vi "Calculate Ball Trajectory.vi"() -> ()   [LabVIEW 2013]
panel:
  in  "Ball Data":T1
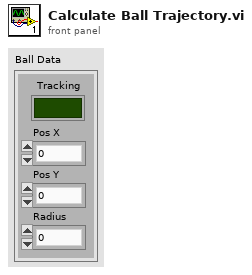
[diagram p1: front panel]
types:
  T1 = cluster{"Tracking":bool, "Pos X":dbl, "Pos Y":dbl, "Radius":dbl}
  T2 = cluster{bool, "Numeric":dbl, "Numeric":dbl, "Numeric":dbl}
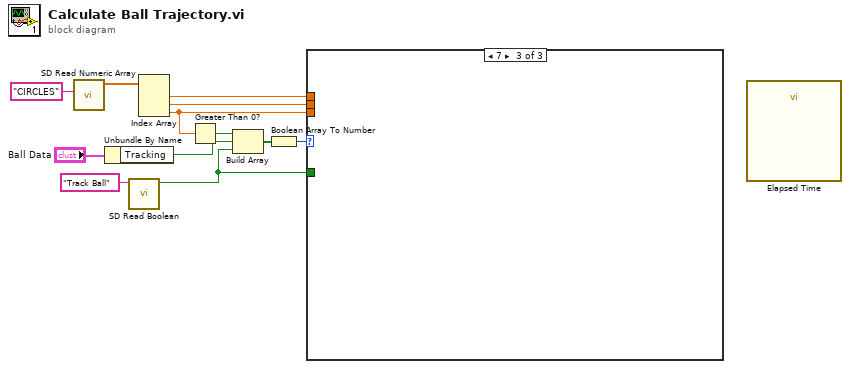
[diagram p0: block diagram]
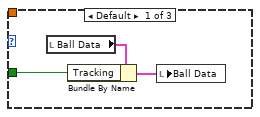
[diagram p2: hidden frame]
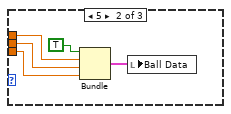
[diagram p3: hidden frame]
diagram:
  n1 = call <vilib>:"SD Read Numeric Array.vi"("Table Prefix"="CIRCLES") -> ("Numeric Array"=w10:dbl[])  [unwired: 8 in, 2 out]
  n2 = Unbundle By Name("Ball Data") -> ("Tracking"=w8:bool)
  n3 = call <vilib>:"SD Read Boolean.vi"("Name"="Track Ball") -> ("Boolean"=w1:bool)  [unwired: 8 in, 2 out]
  n4 = Index Array(array=w10) -> (element #1=w5:dbl, element #2=w4:dbl, element #3=w3:dbl)  [unwired: 3 in]
  n5 = Greater Than 0?(x=w3) -> (x > 0?=w9:bool)
  n6 = Build Array(w9, w8, w1) -> (w6:bool[])
  n7 = Boolean Array To Number(Boolean array=w6) -> (number=w7:u32)
  n8 = case shown="7" w7 {
    tunnel: w5 -> [_ w18 _]
    tunnel: w4 -> [_ w17 _]
    tunnel: w3 -> [_ w16 _]
    tunnel: w1 -> [w15 _ _]
    frame Default {
      n9 = local read "Ball Data"() -> (w13:T1)
      n10 = Bundle By Name(cluster=w13, "Tracking"=w15) -> (w14:T1)
      n11 = local write "Ball Data"(w14) -> ()
    }
    frame 5 {
      n12 = Bundle(TRUE, "Numeric"=w18, "Numeric"=w17, "Numeric"=w16) -> (w20:T2)  [unwired: 1 in]
      n13 = local write "Ball Data"(w20) -> ()
    }
    frame 7 {
    }
  }
  n14 = call "Elapsed Time"() -> ()  [unwired: 12 in, 8 out]
